vi "Mouseover Panel Object.vi"(8 "Error In":errorcluster, 9 "Occurrence":refnum<k4>, 10 "Coords":T1, 11 "Pane Relief Main UI in":refnum<class "Pane Relief Main UI.lvclass">) -> (0 "Error Out":errorcluster, 3 "Pane Relief Main UI out":refnum<class "Pane Relief Main UI.lvclass">)   [LabVIEW 2015, in "Pane Relief Main UI.lvlib" / "Pane Relief Main UI.lvclass"]
uses:
  Pane Relief Main UI.lvclass
  <vilib>/Utility/miscctls.llb/LVPoint32TypeDef.ctl
  Pane Relief Main UI.lvclass/Pane Relief Main UI.ctl
  Classes/Panel Object/Panel Object.lvclass
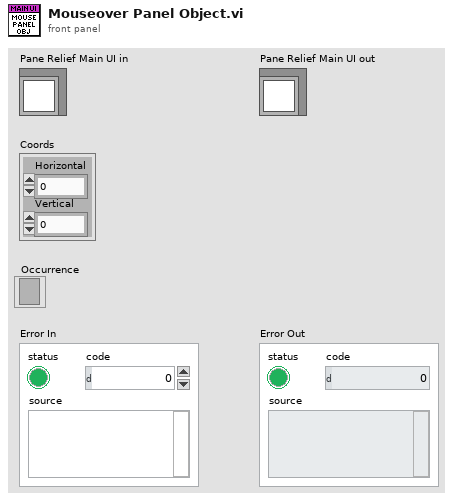
[diagram p1: front panel]
types:
  T1 = typedef "LVPoint32TypeDef.ctl" = cluster{"Horizontal":i32, "Vertical":i32}
  T2 = typedef "Point--Cluster.ctl" = cluster{"Horizontal":i32, "Vertical":i32}
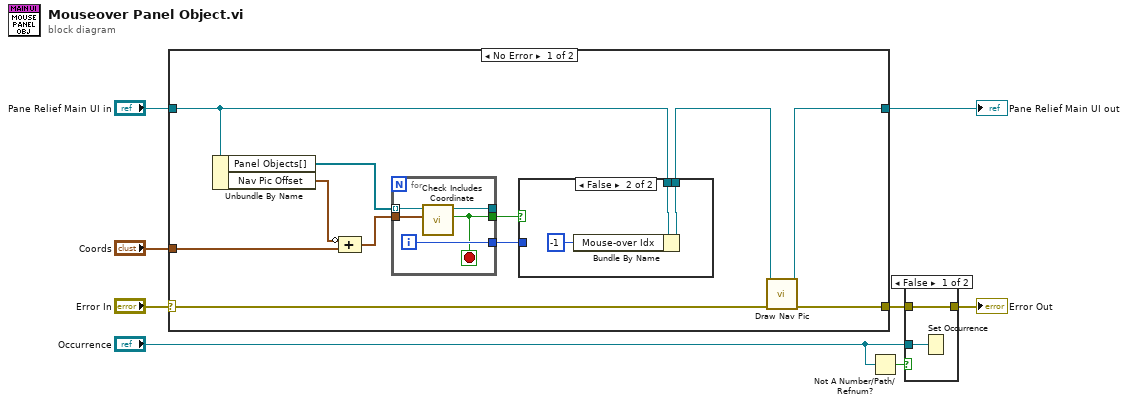
[diagram p0: block diagram]
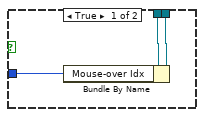
[diagram p3: hidden frame]
diagram:
  n1 = case shown="No Error" "Error In" {
    selector: "Error In" -> [w13 w32]
    tunnel: [w11 w32] -> w2
    tunnel: [w9 w31] -> w7
    tunnel: "Pane Relief Main UI in" -> [w10 w31]
    tunnel: "Coords" -> [w14 _]
    frame No Error {
      n2 = Unbundle By Name(w10) -> ("Panel Objects[]"=w17:refnum<class "Panel Object.lvclass">[], "Nav Pic Offset"=w18:T2)
      n3 = Compound Arithmetic op=ADD(invert w18, w14) -> (w16:T2)
      n4 = for {
        tunnel: [w30] -> _
        tunnel: [w26] -> w19
        tunnel: w17 -> [w29] mode=indexing
        tunnel: w16 -> [w28]
        tunnel: [w27] -> w15
        i -> [w27]
        stop <- w26 stop-if-true
        n5 = call-dynamic "Check Includes Coordinate.vi"("Coordinate"=w28, "Panel Object in"=w29) -> ("Included?"=w26:bool, "Panel Object out"=w30:refnum<class "Panel Object.lvclass">)  [unwired: 7 in, 1 out]
      }
      n6 = case shown="False" w19 {
        tunnel: [w22 w25] -> w12
        tunnel: w10 -> [w21 w24]
        tunnel: w15 -> [w20 _]
        frame True {
          n7 = Bundle By Name(cluster=w21, "Mouse-over Idx"=w20) -> (w22:refnum<class "Pane Relief Main UI.lvclass">)
        }
        frame False {
          n8 = Bundle By Name(cluster=w24, "Mouse-over Idx"=-1 ("UI Selections.Mouse-over Idx")) -> (w25:refnum<class "Pane Relief Main UI.lvclass">)
        }
      }
      n9 = call-dynamic "Draw Nav Pic.vi"("Error In"=w13, "Pane Relief Main UI in"=w12) -> ("Error Out"=w11:errorcluster, "Pane Relief Main UI out"=w9:refnum<class "Pane Relief Main UI.lvclass">)  [unwired: 8 in]
    }
    frame Error {
    }
  }
  "Pane Relief Main UI out" <- w7
  n10 = Not A Number/Path/Refnum?(number/path/refnum="Occurrence") -> (NaN/Path/Refnum?=w3:bool)
  n11 = case shown="False" w3 {
    tunnel: "Occurrence" -> [w34 _]
    tunnel: w2 -> [w33 w35]
    tunnel: [w33 w35] -> w1
    frame False {
      n12 = Set Occurrence(w34) -> ()
    }
    frame True {
    }
  }
  "Error Out" <- w1
